vi "2401 Wire.vi"(9 "4-wire":bool) -> ()   [LabVIEW 2009]
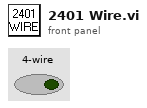
[diagram p1: front panel]
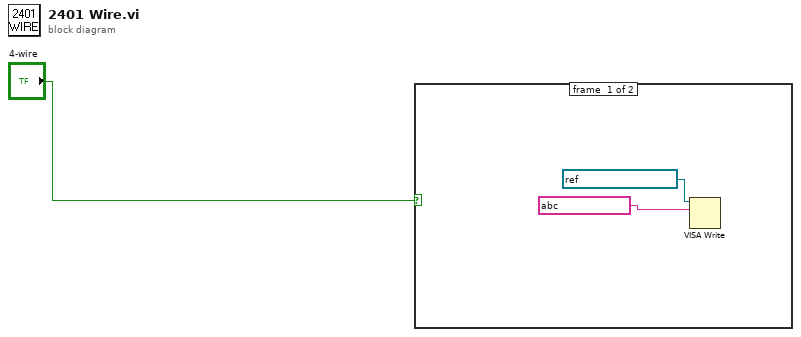
[diagram p0: block diagram]
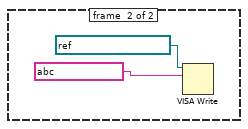
[diagram p2: hidden frame]
diagram:
  n1 = case shown="True" "4-wire" {
    frame #0 {
      n2 = VISA Write(VISA resource name=refnum<visa-resource-name> ?, write buffer=string ?) -> ()  [unwired: 1 in, 3 out]
    }
    frame #1 {
      n3 = VISA Write(VISA resource name=refnum<visa-resource-name> ?, write buffer=string ?) -> ()  [unwired: 1 in, 3 out]
    }
  }
